vi "Subscriber-1.vi"() -> ()   [LabVIEW 2019]
uses:
  <vilib>/Distrio/LabbitMQ/Channel/exchange_type_enum.ctl
  <vilib>/Distrio/LabbitMQ/Connection/Connection.lvclass
  <vilib>/Distrio/LabbitMQ/Connection/connection_parameters_cluster.ctl
  <vilib>/Distrio/LabbitMQ/Channel/Channel.lvclass
  <vilib>/Distrio/LabbitMQ/Queue/Queue.lvclass
panel:
  out "Received Message":string
  in  "Subscribe":bool
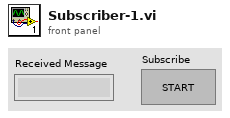
[diagram p1: front panel]
types:
  T1 = typedef "Connection.lvclass/connection_parameters_cluster.ctl" = cluster{"host name":string, "port":i32, "user name":string, "password":string, "virtual host":string}
  T2 = typedef "Channel.lvclass/exchange_type_enum.ctl" = enum16{"direct", "topic", "fanout", "headers"}
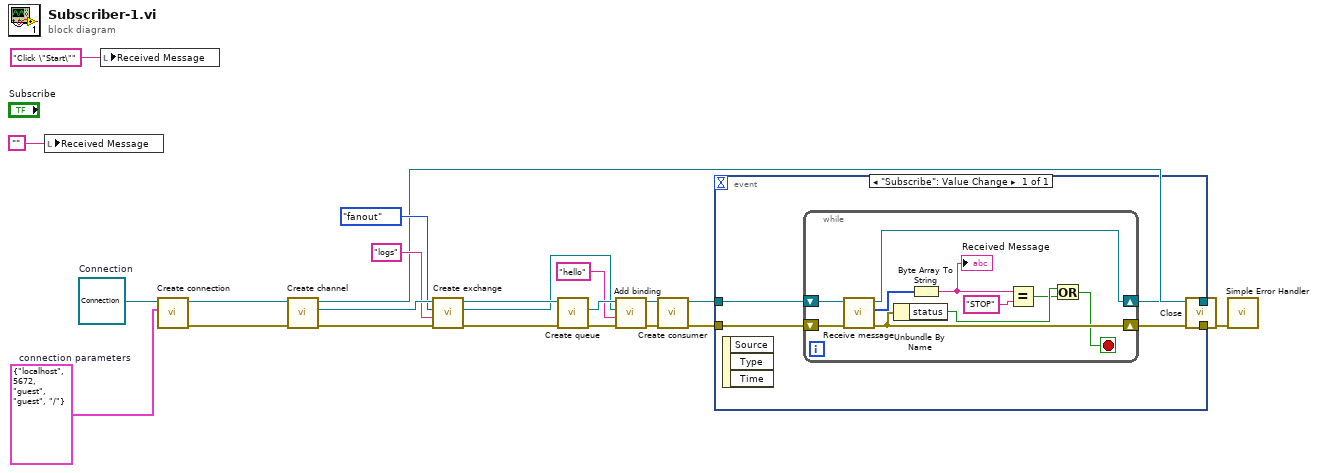
[diagram p0: block diagram]
diagram:
  w8 = T1 {"host name"="localhost", "port"=5672, "user name"="guest", "password"="guest", "virtual host"="/"}  # connection parameters
  w9 = refnum<class "Connection.lvclass"> refnum  # Connection
  n1 = local write "Received Message"("") -> ()
  n2 = local write "Received Message"("Click \"Start\"") -> ()
  n3 = call <vilib>:"Create connection.vi"("connection parameters"=w8, "Connection in"=w9) -> ("error out"=w22:errorcluster, "Connection out"=w23:refnum<class "Connection.lvclass">)  [unwired: 8 in]
  n4 = call <vilib>:"Create channel.vi"("error in (no error)"=w22, "Connection in"=w23) -> ("error out"=w21:errorcluster, "channel"=w20:refnum<class "Channel.lvclass">, "Connection out"=w7:refnum<class "Connection.lvclass">)  [unwired: 7 in]
  n5 = call <vilib>:"Create exchange.vi"("error in (no error)"=w21, "exchange name"="logs", "exchange type"=exchange_type_enum."fanout" ("binding"), "Channel in"=w20) -> ("error out"=w19:errorcluster, "Exchange.lvclass"=w15:refnum<class "Exchange.lvclass">, "Channel out"=w18:refnum<class "Channel.lvclass">)  [unwired: 5 in]
  n6 = call <vilib>:"Create queue.vi"("error in (no error)"=w19, "Channel in"=w18) -> ("error out"=w17:errorcluster, "Queue.lvclass"=w16:refnum<class "Queue.lvclass">)  [unwired: 7 in, 1 out]
  n7 = call <vilib>:"Add binding.vi"("error in (no error)"=w17, "binding key"="hello" ("routing key"), "Exchange.lvclass"=w15, "Consumer in"=w16) -> ("error out"=w13:errorcluster, "Consumer out"=w12:refnum<class "Queue.lvclass">)  [unwired: 6 in]
  n8 = call <vilib>:"Create consumer.vi"("error in (no error)"=w13, "Queue in"=w12) -> ("error out"=w4:errorcluster, "Queue out"=w5:refnum<class "Queue.lvclass">)  [unwired: 8 in]
  n9 = event shown="[0] \"Subscribe\": Value Change" {
    selector: _ -> [_]
    dyn-events: _ -> [_]
    timeout: _ -> [_]
    tunnel: w5 -> [w27]
    tunnel: w4 -> [w26]
    tunnel: [w25] -> _
    tunnel: [w24] -> w3
    event "Subscribe": Value Change {
      n10 = event-data() -> ()  [unwired: 1 in, 3 out]
      n11 = while {
        shift-right: [w34] -> w25
        shift-left: w27 -> [w36]
        shift-right: [w30] -> w24
        shift-left: w26 -> [w35]
        stop <- w29 stop-if-true
        n12 = call <vilib>:"Receive message.vi"("error in (no error)"=w35, "Consumer in"=w36) -> ("error out"=w30:errorcluster, "message body"=w37:u8[], "Consumer out"=w34:refnum<class "Queue.lvclass">)  [unwired: 4 in, 3 out]
        n13 = Unbundle By Name(w30) -> ("status"=w31:bool)
        n14 = Byte Array To String(unsigned byte array=w37) -> (string=w32:string)
        "Received Message" <- w32
        n15 = Equal?(x=w32, y="STOP") -> (x = y?=w28:bool)
        n16 = Or(x=w31, y=w28) -> (x .or. y?=w29:bool)
      }
    }
  }
  n17 = call <vilib>:"Close.vi"("error in (no error)"=w3, "Connection in"=w7) -> ("error out"=w6:errorcluster)  [unwired: 8 in, 1 out]
  n18 = call <vilib>:"Simple Error Handler.vi"("error in (no error)"=w6) -> ()  [unwired: 4 in, 5 out]
